vi "主程序.vi"() -> ()   [LabVIEW 2013]
panel:
  out "人血量":i32(slide) scale=0.0..200.0
  in  "停止":bool
  in  "怪兽 2":bool=TRUE
  in  "怪兽":bool
  in  "枚举 2":enum16{"初始化", "后退", "施法", "出击"}(ring)
  in  "12":bool
  in  "7":bool
  in  "4":bool
  in  "11":bool
  in  "8":bool
  in  "10":bool
  in  "3":bool
  in  "9":bool
  in  "2":bool
  in  "6":bool
  in  "13":bool
  in  "5":bool
  in  "1":bool
  in  "枚举":enum16{"敌方攻击", "时间条状态"}(ring)
  out "怪物血量":i32(slide) scale=0.0..400.0
  out "我方行动值":i32
  out "敌方行动值":i32
  in  "怪物速度":i32
  in  "人速度":i32
  out "怪物行动":i32(slide) scale=0.0..100.0
  out "人行动":i32(slide) scale=0.0..100.0
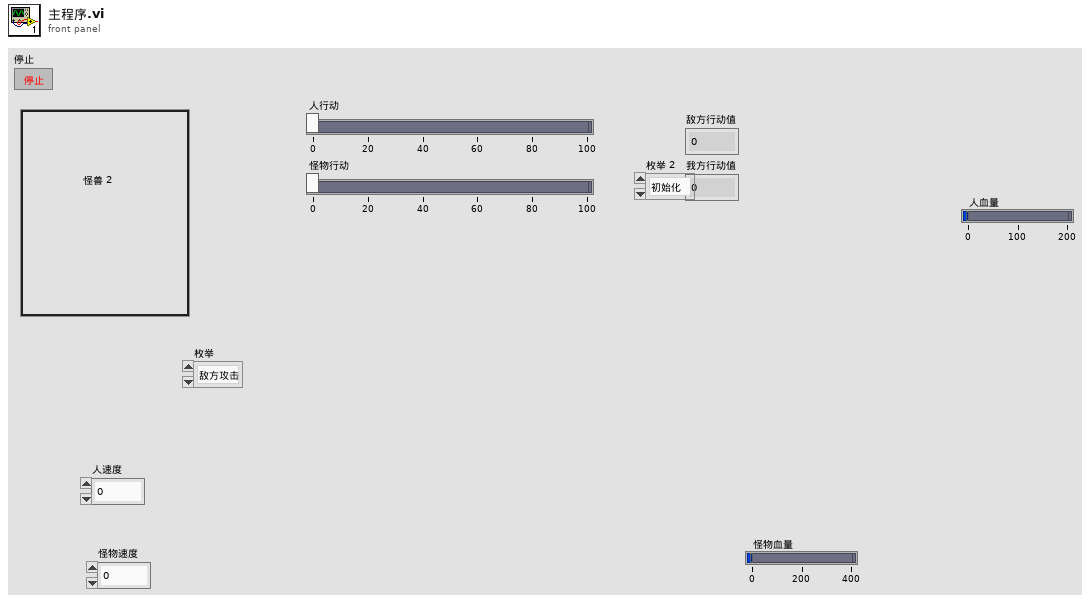
[diagram p1: front panel]
types:
  T1 = cluster{bool, bool, bool, bool, bool, bool, bool, bool, bool, bool, bool, bool, bool}
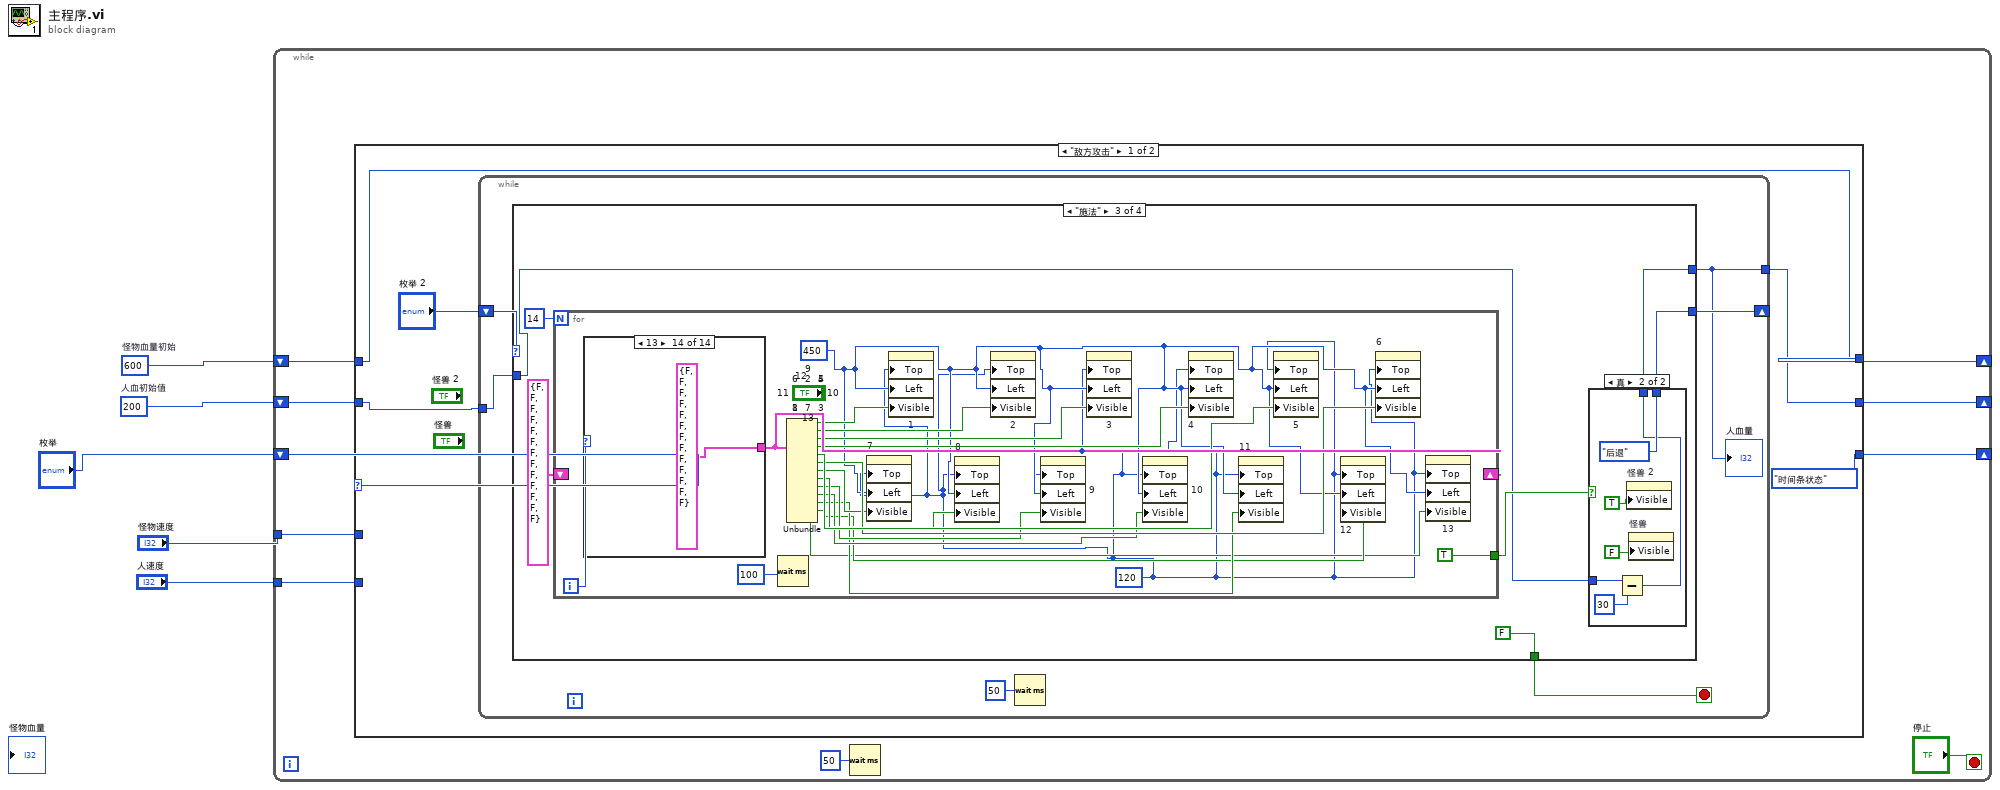
[diagram p0: block diagram]
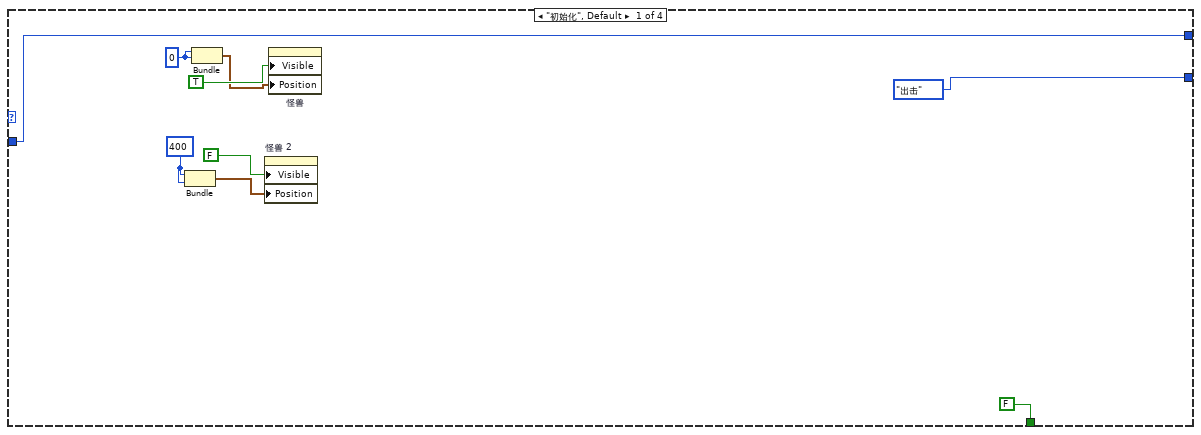
[diagram p2: hidden frame]
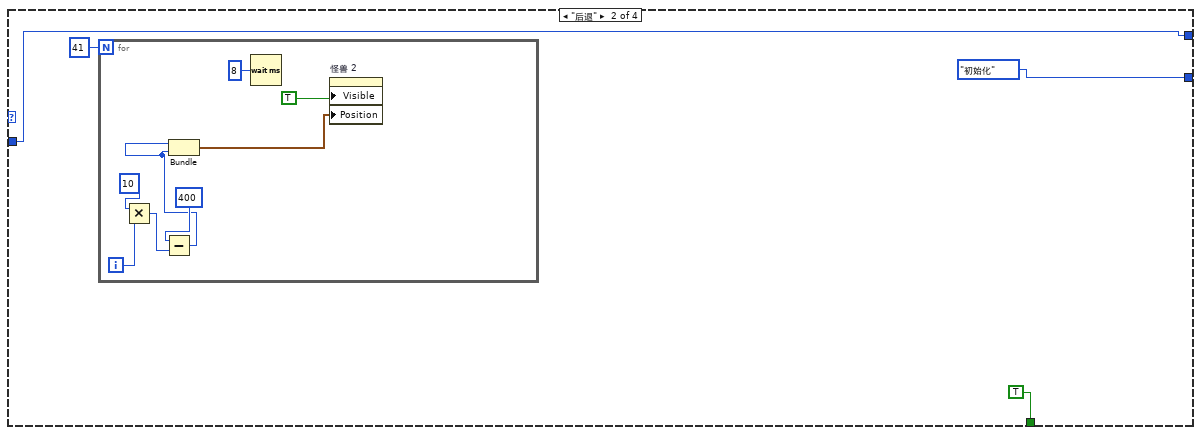
[diagram p3: hidden frame]
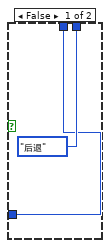
[diagram p4: hidden frame]
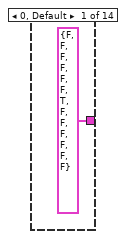
[diagram p5: hidden frame]
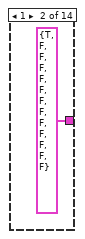
[diagram p6: hidden frame]
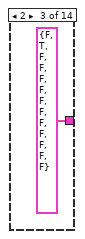
[diagram p7: hidden frame]
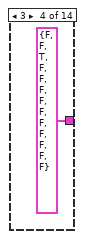
[diagram p8: hidden frame]
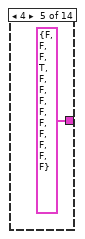
[diagram p9: hidden frame]
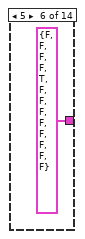
[diagram p10: hidden frame]
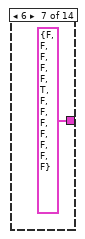
[diagram p11: hidden frame]
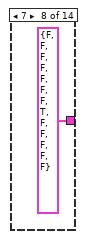
[diagram p12: hidden frame]
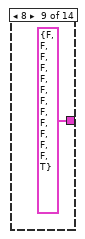
[diagram p13: hidden frame]
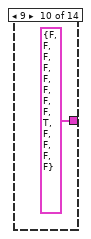
[diagram p14: hidden frame]
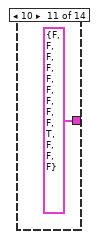
[diagram p15: hidden frame]
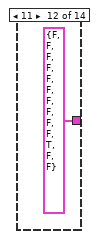
[diagram p16: hidden frame]
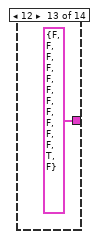
[diagram p17: hidden frame]
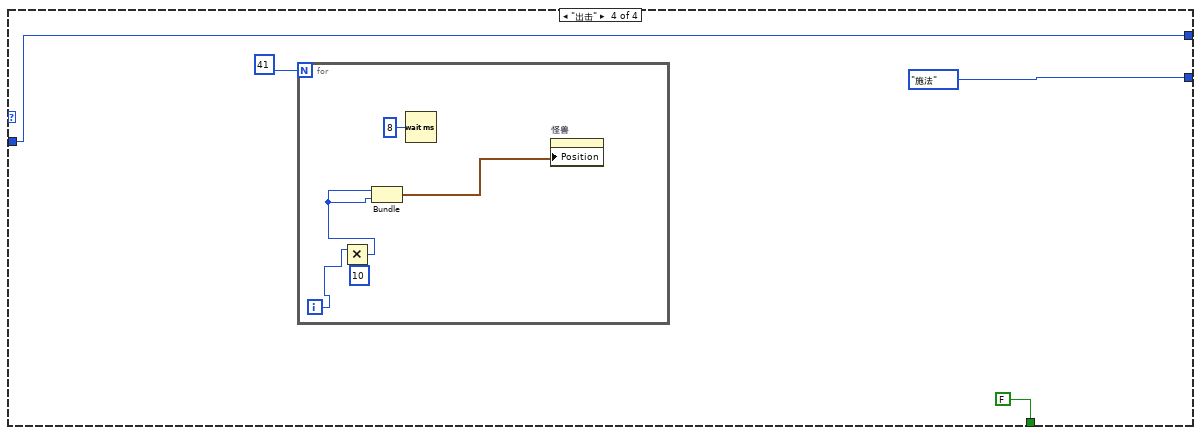
[diagram p18: hidden frame]
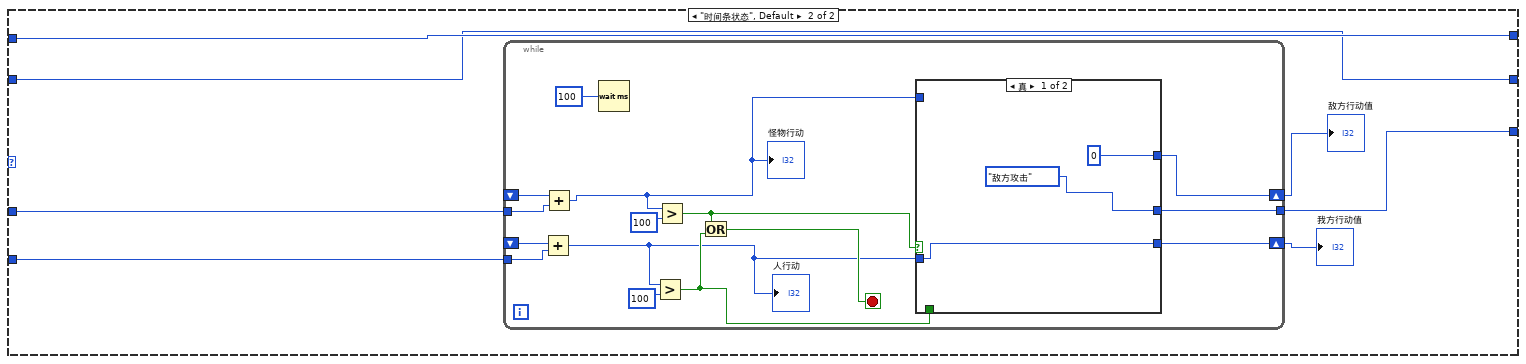
[diagram p19: hidden frame]
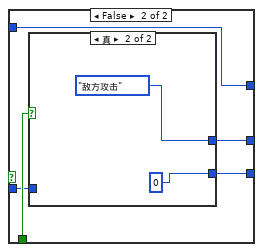
[diagram p20: hidden frame]
diagram:
  w2 = 200  # 人血初始值
  w3 = 600  # 怪物血量初始
  n1 = while {
    tunnel: "怪物速度" -> [w15]
    tunnel: "人速度" -> [w14]
    shift-right: [w10] -> _
    shift-left: w3 -> [w12]
    shift-right: [w8] -> _
    shift-left: w2 -> [w11]
    shift-right: [w9] -> _
    shift-left: "枚举" -> [w13]
    stop <- "停止" stop-if-true
    n2 = case shown="\"敌方攻击\"" w13 {
      tunnel: w15 -> [_ w111]
      tunnel: w14 -> [_ w110]
      tunnel: [enum16{"敌方攻击", "时间条状态"}."时间条状态" ("枚举") w109] -> w9
      tunnel: w12 -> [w16 w108]
      tunnel: w11 -> [w18 w107]
      tunnel: [w16 w108] -> w10
      tunnel: [w17 w107] -> w8
      frame "敌方攻击" {
        n3 = while {
          shift-right: [w25] -> _
          shift-left: "枚举 2" -> [w26]
          tunnel: w18 -> [w23]
          tunnel: [w21] -> w17
          stop <- w24 stop-if-true
          n4 = case shown="\"施法\"" w26 {
            tunnel: [enum16{"初始化", "后退", "施法", "出击"}."出击" ("枚举") enum16{"初始化", "后退", "施法", "出击"}."初始化" ("枚举") w51 enum16{"初始化", "后退", "施法", "出击"}."施法" ("枚举")] -> w25
            tunnel: [FALSE TRUE FALSE FALSE] -> w24
            tunnel: w23 -> [w27 w37 w49 w97]
            tunnel: [w27 w37 w48 w97] -> w21
            frame "初始化", Default {
              w34 = 400
              w35 = 0
              n5 = Bundle(w34, w34) -> (w30:cluster{i32, i32})  [unwired: 1 in]
              n6 = Bundle(w35, w35) -> (w31:cluster{i32, i32})  [unwired: 1 in]
              n7 = property on="怪兽 2" class="Bool"("Visible"=FALSE, "Position"=w30) -> ()  [unwired: 2 in, 2 out]
              n8 = property on="怪兽" class="Bool"("Visible"=TRUE, "Position"=w31) -> ()  [unwired: 2 in, 2 out]
            }
            frame "后退" {
              n9 = for {
                N: 41 -> [_]
                i -> [w43]
                n10 = Multiply(x=10, y=w43) -> (x*y=w41:i32)
                n11 = Subtract(x=400, y=w41) -> (x-y=w40:i32)
                n12 = Bundle(w40, w40) -> (w45:cluster{i32, i32})  [unwired: 1 in]
                n13 = Wait (ms)(milliseconds to wait=u32 8 ("等待时间（毫秒）")) -> ()  [unwired: 1 out]
                n14 = property on="怪兽 2" class="Bool"("Visible"=TRUE, "Position"=w45) -> ()  [unwired: 2 in, 2 out]
              }
            }
            frame "施法" {
              n15 = for {
                N: 14 -> [_]
                shift-right: [w80] -> _
                shift-left: T1 {FALSE, FALSE, FALSE, FALSE, FALSE, FALSE, FALSE, FALSE, FALSE, FALSE, FALSE, FALSE, FALSE} -> [_]
                tunnel: [TRUE] -> w52
                i -> [w81]
                w65 = 120
                w66 = 450
                n16 = case shown="13" w81 {
                  tunnel: [T1 {FALSE, FALSE, FALSE, FALSE, FALSE, FALSE, TRUE, FALSE, FALSE, FALSE, FALSE, FALSE, FALSE} T1 {TRUE, FALSE, FALSE, FALSE, FALSE, FALSE, FALSE, FALSE, FALSE, FALSE, FALSE, FALSE, FALSE} T1 {FALSE, TRUE, FALSE, FALSE, FALSE, FALSE, FALSE, FALSE, FALSE, FALSE, FALSE, FALSE, FALSE} T1 {FALSE, FALSE, TRUE, FALSE, FALSE, FALSE, FALSE, FALSE, FALSE, FALSE, FALSE, FALSE, FALSE} T1 {FALSE, FALSE, FALSE, TRUE, FALSE, FALSE, FALSE, FALSE, FALSE, FALSE, FALSE, FALSE, FALSE} T1 {FALSE, FALSE, FALSE, FALSE, TRUE, FALSE, FALSE, FALSE, FALSE, FALSE, FALSE, FALSE, FALSE} T1 {FALSE, FALSE, FALSE, FALSE, FALSE, TRUE, FALSE, FALSE, FALSE, FALSE, FALSE, FALSE, FALSE} T1 {FALSE, FALSE, FALSE, FALSE, FALSE, FALSE, FALSE, TRUE, FALSE, FALSE, FALSE, FALSE, FALSE} T1 {FALSE, FALSE, FALSE, FALSE, FALSE, FALSE, FALSE, FALSE, FALSE, FALSE, FALSE, FALSE, TRUE} T1 {FALSE, FALSE, FALSE, FALSE, FALSE, FALSE, FALSE, FALSE, TRUE, FALSE, FALSE, FALSE, FALSE} T1 {FALSE, FALSE, FALSE, FALSE, FALSE, FALSE, FALSE, FALSE, FALSE, TRUE, FALSE, FALSE, FALSE} T1 {FALSE, FALSE, FALSE, FALSE, FALSE, FALSE, FALSE, FALSE, FALSE, FALSE, TRUE, FALSE, FALSE} T1 {FALSE, FALSE, FALSE, FALSE, FALSE, FALSE, FALSE, FALSE, FALSE, FALSE, FALSE, TRUE, FALSE} T1 {FALSE, FALSE, FALSE, FALSE, FALSE, FALSE, FALSE, FALSE, FALSE, FALSE, FALSE, FALSE, FALSE}] -> w80
                  frame 0, Default {
                  }
                  frame 1 {
                  }
                  frame 2 {
                  }
                  frame 3 {
                  }
                  frame 4 {
                  }
                  frame 5 {
                  }
                  frame 6 {
                  }
                  frame 7 {
                  }
                  frame 8 {
                  }
                  frame 9 {
                  }
                  frame 10 {
                  }
                  frame 11 {
                  }
                  frame 12 {
                  }
                  frame 13 {
                  }
                }
                n17 = Wait (ms)(milliseconds to wait=100) -> ()  [unwired: 1 out]
                n18 = Unbundle(w80) -> (w79:bool, w78:bool, w77:bool, w76:bool, w75:bool, w74:bool, w73:bool, w72:bool, w71:bool, w70:bool, w69:bool, w68:bool, w67:bool)
                n19 = property on="7" class="Bool"("Top"=w65, "Left"=w66, "Visible"=w73) -> ()  [unwired: 2 in, 2 out]
                n20 = property on="1" class="Bool"("Top"=w65, "Left"=w66, "Visible"=w79) -> ()  [unwired: 2 in, 2 out]
                n21 = property on="8" class="Bool"("Top"=w65, "Left"=w66, "Visible"=w72) -> ()  [unwired: 2 in, 2 out]
                n22 = property on="2" class="Bool"("Top"=w65, "Left"=w66, "Visible"=w78) -> ()  [unwired: 2 in, 2 out]
                n23 = property on="9" class="Bool"("Top"=w65, "Left"=w66, "Visible"=w71) -> ()  [unwired: 2 in, 2 out]
                n24 = property on="3" class="Bool"("Top"=w65, "Left"=w66, "Visible"=w77) -> ()  [unwired: 2 in, 2 out]
                n25 = property on="10" class="Bool"("Top"=w65, "Left"=w66, "Visible"=w70) -> ()  [unwired: 2 in, 2 out]
                n26 = property on="4" class="Bool"("Top"=w65, "Left"=w66, "Visible"=w76) -> ()  [unwired: 2 in, 2 out]
                n27 = property on="11" class="Bool"("Top"=w65, "Left"=w66, "Visible"=w69) -> ()  [unwired: 2 in, 2 out]
                n28 = property on="5" class="Bool"("Top"=w65, "Left"=w66, "Visible"=w75) -> ()  [unwired: 2 in, 2 out]
                n29 = property on="12" class="Bool"("Top"=w65, "Left"=w66, "Visible"=w68) -> ()  [unwired: 2 in, 2 out]
                n30 = property on="6" class="Bool"("Top"=w65, "Left"=w66, "Visible"=w74) -> ()  [unwired: 2 in, 2 out]
                n31 = property on="13" class="Bool"("Top"=w65, "Left"=w66, "Visible"=w67) -> ()  [unwired: 2 in, 2 out]
              }
              n32 = case shown="真" w52 {
                tunnel: [enum16{"初始化", "后退", "施法", "出击"}."后退" ("枚举") enum16{"初始化", "后退", "施法", "出击"}."后退" ("枚举")] -> w51
                tunnel: w49 -> [w55 w59]
                tunnel: [w55 w57] -> w48
                frame False {
                }
                frame True {
                  n33 = Subtract(x=w59, y=30) -> (x-y=w57:i32)
                  n34 = property on="怪兽 2" class="Bool"("Visible"=TRUE) -> ()  [unwired: 2 in, 2 out]
                  n35 = property on="怪兽" class="Bool"("Visible"=FALSE) -> ()  [unwired: 2 in, 2 out]
                }
              }
            }
            frame "出击" {
              n36 = for {
                N: 41 -> [_]
                i -> [w102]
                n37 = Multiply(x=w102, y=10) -> (x*y=w100:i32)
                n38 = Bundle(w100, w100) -> (w103:cluster{i32, i32})  [unwired: 1 in]
                n39 = Wait (ms)(milliseconds to wait=u32 8 ("等待时间（毫秒）")) -> ()  [unwired: 1 out]
                n40 = property on="怪兽" class="Bool"("Position"=w103) -> ()  [unwired: 2 in, 2 out]
              }
            }
          }
          "人血量" <- w21
          n41 = Wait (ms)(milliseconds to wait=u32 50 ("等待时间（毫秒）")) -> ()  [unwired: 1 out]
        }
      }
      frame "时间条状态", Default {
        n42 = while {
          shift-right: [w112] -> w106
          shift-left: _ -> [w123]
          shift-right: [w113] -> w105
          shift-left: _ -> [w125]
          tunnel: w111 -> [w126]
          tunnel: w110 -> [w124]
          tunnel: [w117] -> w109
          stop <- w120 stop-if-true
          n43 = Add(x=w123, y=w124) -> (x+y=w115:i32)
          "人行动" <- w115
          n44 = Add(x=w125, y=w126) -> (x+y=w116:i32)
          "怪物行动" <- w116
          n45 = Wait (ms)(milliseconds to wait=100) -> ()  [unwired: 1 out]
          n46 = Greater?(x=w115, y=100) -> (0:w118:bool)
          n47 = Greater?(x=w116, y=100) -> (0:w119:bool)
          n48 = Or(x=w119, y=w118) -> (x .or. y?=w120:bool)
          n49 = case shown="真" w119 {
            tunnel: [enum16{"敌方攻击", "时间条状态"}."敌方攻击" ("枚举") w134] -> w117
            tunnel: w118 -> [_ w133]
            tunnel: [0 w132] -> w113
            tunnel: w116 -> [_ w132]
            tunnel: [w128 w131] -> w112
            tunnel: w115 -> [w128 w130]
            frame True {
            }
            frame False {
              n50 = case shown="真" w133 {
                tunnel: [enum16{"敌方攻击", "时间条状态"}."时间条状态" ("枚举") enum16{"敌方攻击", "时间条状态"}."敌方攻击" ("枚举")] -> w134
                tunnel: [w136 0] -> w131
                tunnel: w130 -> [w136 _]
                frame False {
                }
                frame True {
                }
              }
            }
          }
        }
        "敌方行动值" <- w105
        "我方行动值" <- w106
      }
    }
    n51 = Wait (ms)(milliseconds to wait=u32 50 ("等待时间（毫秒）")) -> ()  [unwired: 1 out]
  }
